vi "dfd_Decide NStage Interpolated Factors.vi"(6 "fs in [Hz]":dbl, 8 "error in (no error)":errorcluster, 11 "multirate filters in":T1[](array[typedef]) {"mMRate_SumWl" min=1 max=32 step=1; "mMRate_InputIwl" min=1 max=32 step=1; "mMRate_GainWl" min=1 max=32 step=1; "mMRate_OutputWl" min=1 max=32 step=1; "mMRate_InputWl" min=1 max=32 step=1; "mMRate_CoefWl" min=1 max=32 step=1; "mMRate_Mode" items=["Default"=-1, "No Rate Change"=0, "Interpolation"=1, "Decimation"=2, "Interpolated"=3, "Rational"=4]}) -> (0 "error out":errorcluster, 1 "interpolated factors":i32[](array[numeric]), 2 "no overall?":bool, 3 "dup multirate filters in":T1[](array[typedef]) {"mMRate_SumWl" min=1 max=32 step=1; "mMRate_InputIwl" min=1 max=32 step=1; "mMRate_GainWl" min=1 max=32 step=1; "mMRate_OutputWl" min=1 max=32 step=1; "mMRate_InputWl" min=1 max=32 step=1; "mMRate_CoefWl" min=1 max=32 step=1; "mMRate_Mode" items=["Default"=-1, "No Rate Change"=0, "Interpolation"=1, "Decimation"=2, "Interpolated"=3, "Rational"=4]}, 4 "equivalent fs":dbl)   [LabVIEW 2017, in "NI_DigFilterLicensed.lvlib"]
uses:
  <vilib>/addons/Digital Filter Design/NI_DigFilterLicensed.lvlib
  <vilib>/addons/Digital Filter Design/_Objects.llb/DFD Multirate Filter Obj.ctl
  <vilib>/addons/Digital Filter Design/_Objects.llb/DFD Multirate Mode.ctl
  <vilib>/addons/Digital Filter Design/_Objects.llb/DFD Coef Norm Type.ctl
  <vilib>/addons/Digital Filter Design/_Objects.llb/DFD Round-off Mode.ctl
  <vilib>/addons/Digital Filter Design/_Objects.llb/DFD FXP MRate Multiply Mode.ctl
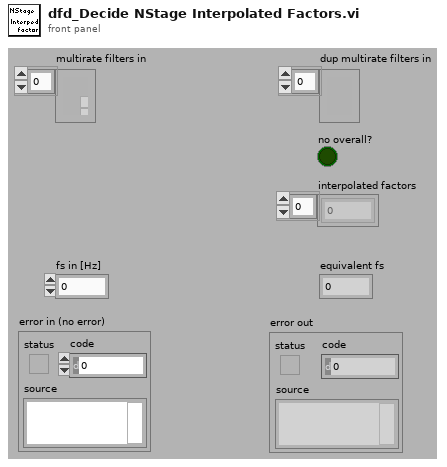
[diagram p1: front panel]
types:
  T1 = typedef "NI_DigFilterLicensed.lvlib/DFD Multirate Filter Obj.ctl" = cluster{"mMRate_Structure":enum16{"CIC", "FIR", "IIR", "Lattice"}, "mMRate_Mode":T2, "mMRate_Factor":i32, "mMRate_FIRParams":cluster{"mMRate_FIR_H":dbl[], "mMRate_FIR_IsNyquist?":bool, "mMRate_FIR_IsSymmetric?":bool}, "mMRate_CICParams":cluster{"mMRate_CIC_#Stage":i32, "mMRate_CIC_Lag":i32, "mMRate_CIC_Type":enum16{"Lowpass", "Highpass"}}, "mMRate_Order":i32, "mMRate_Version":string, "mMRate_Comments":string, "mMRate_RationalFactor":cluster{"mMRate_L":i32, "mMRate_M":i32}, "mMRate_Fs":dbl, "mMRate_Quantized?":bool, "mMRate_QFilterGain":dbl, "mMRate_CoefWl":i16, "mMRate_Scaling":cluster{"mMRate_ScaleByPowerOf2?":bool, "mMRate_ScaleType":T3}, "mMRate_InputWl":i16, "mMRate_OutputWl":i16, "mMRate_OutputMode":T4, "mMRate_MultMode":T5, "mMRate_BitPruning":bool, "mMRate_GainWl":i16, "mMRate_OutputFwl":i16, "mMRate_SumIwl":i16, "mMRate_InputIwl ":i16, "mMRate_SumWl":i16, "mMRate_CoefIwl":i16}
  T2 = typedef "NI_DigFilterLicensed.lvlib/DFD Multirate Mode.ctl" = i16
  T3 = typedef "NI_DigFilterLicensed.lvlib/DFD Coef Norm Type.ctl" = enum16{"No Norm", "Time Domain 1-Norm", "Time Domain 2-Norm", "Time Domain Inf-Norm"}
  T4 = typedef "NI_DigFilterLicensed.lvlib/DFD Round-off Mode.ctl" = enum16{"Nearest", "Truncation"}
  T5 = typedef "NI_DigFilterLicensed.lvlib/DFD FXP MRate Multiply Mode.ctl" = enum16{"Truncated", "Full"}
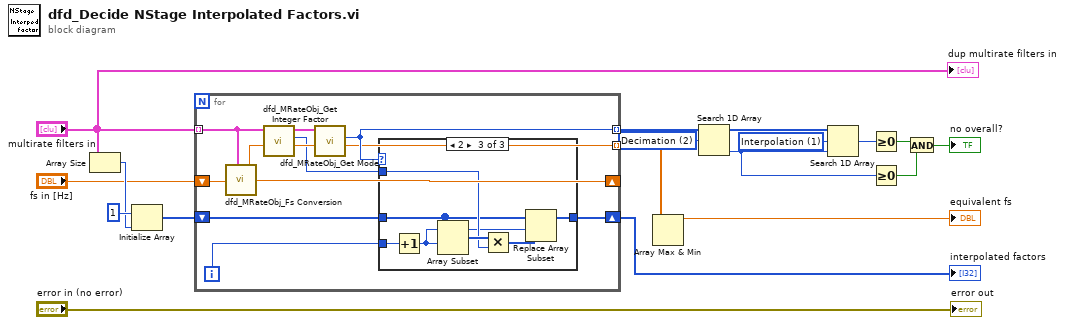
[diagram p0: block diagram]
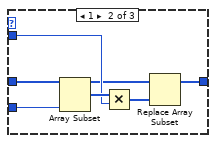
[diagram p3: hidden frame]
diagram:
  w11 = T2 1 items=["Default"=-1, "No Rate Change"=0, "Interpolation"=1, "Decimation"=2, "Interpolated"=3] ("element")
  w13 = T2 2 items=["Default"=-1, "No Rate Change"=0, "Interpolation"=1, "Decimation"=2, "Interpolated"=3] ("element")
  n1 = Array Size(array="multirate filters in") -> (size(s)=w16:i32)
  n2 = Initialize Array(1, w16) -> (w15:i32[])
  n3 = for {
    tunnel: "multirate filters in" -> [w19] mode=indexing
    shift-right: [w25] -> w14
    shift-left: w15 -> [w27]
    tunnel: [w24] -> w12 mode=indexing
    shift-right: [w23] -> _
    shift-left: "fs in [Hz]" -> [w20]
    tunnel: [w21] -> w3 mode=indexing
    i -> [w26]
    n4 = call <vilib>:"dfd_MRateObj_Fs Conversion.vi"("multirate filter"=w19, "fsin"=w20) -> ("filter fs"=w21:dbl, "fsout"=w23:dbl)  [unwired: 4 out]
    n5 = call <vilib>:"dfd_MRateObj_Get Integer Factor.vi"("multirate filter in"=w19) -> ("factor"=w18:i32, "dup multirate filter"=w22:T1)  [unwired: 9 out]
    n6 = call <vilib>:"dfd_MRateObj_Get Mode.vi"("multirate filter in"=w22) -> ("mode"=w24:T2)  [unwired: 10 out]
    n7 = case shown="2" w24 {
      tunnel: w18 -> [_ w33 w39]
      tunnel: w27 -> [w28 w32 w38]
      tunnel: w26 -> [_ w29 w41]
      tunnel: [w28 w31 w36] -> w25
      frame 0, Default {
      }
      frame 1 {
        n8 = Array Subset(array=w32, length=w29) -> (w34:i32[])  [unwired: 1 in]
        n9 = Multiply(x=w34, y=w33) -> (x*y=w30:i32[])
        n10 = Replace Array Subset(array=w32, new element=w30) -> (w31:i32[])  [unwired: 1 in]
      }
      frame 2 {
        n11 = Increment(x=w41) -> (x+1=w37:i32)
        n12 = Array Subset(array=w38, index=w37) -> (w40:i32[])  [unwired: 1 in]
        n13 = Multiply(x=w40, y=w39) -> (x*y=w35:i32[])
        n14 = Replace Array Subset(array=w38, new element=w35, index=w37) -> (w36:i32[])
      }
    }
  }
  "interpolated factors" <- w14
  n15 = Array Max & Min(array=w3) -> (max value=→"equivalent fs":dbl)  [unwired: 3 out]
  n16 = Search 1D Array(1D array=w12, element=w13) -> (index of element=w9:i32)  [unwired: 1 out]
  n17 = Search 1D Array(1D array=w12, element=w11, start index (0)=w9) -> (index of element=w10:i32)
  n18 = Greater Or Equal To 0?(x=w10) -> (x >= 0?=w8:bool)
  n19 = Greater Or Equal To 0?(x=w9) -> (x >= 0?=w7:bool)
  n20 = And(x=w8, y=w7) -> (x .and. y?=→"no overall?":bool)
  "dup multirate filters in" <- "multirate filters in"
  "error out" <- "error in (no error)"
